vi "SFC_Get Hang Carton.vi"(8 "error in (no error)":errorcluster caption="错误输入（无错误）", 11 "Traceability 引用句柄":refnum<k24>) -> (0 "error out":errorcluster caption="错误输出", 2 ".NET:System.Data.DataSet":T1={"CaseSensitive"=FALSE, "Container"=refnum, "DataSetName"="", "DefaultViewManager"=refnum, "DesignMode"=FALSE, "EnforceConstraints"=FALSE, "ExtendedProperties"=refnum, "HasErrors"=FALSE, "IsInitialized"=FALSE, "Locale"=refnum, "Namespace"="", "Prefix"="", "Relations"=refnum, "RemotingFormat"=0, "SchemaSerializationMode"=1, "Site"=refnum, "Tables"=refnum} {"SchemaSerializationMode" items=["IncludeSchema"=1, "ExcludeSchema"=2]; "RemotingFormat" items=["Xml", "Binary"]}, 3 "Traceability 引用句柄输出":refnum<k24>)   [LabVIEW 2014, in "Traceability.lvlib"]
uses:
  D:/webservice/Traceability.dll
  Traceability.dll
  System.Data
  Traceability.lvlib
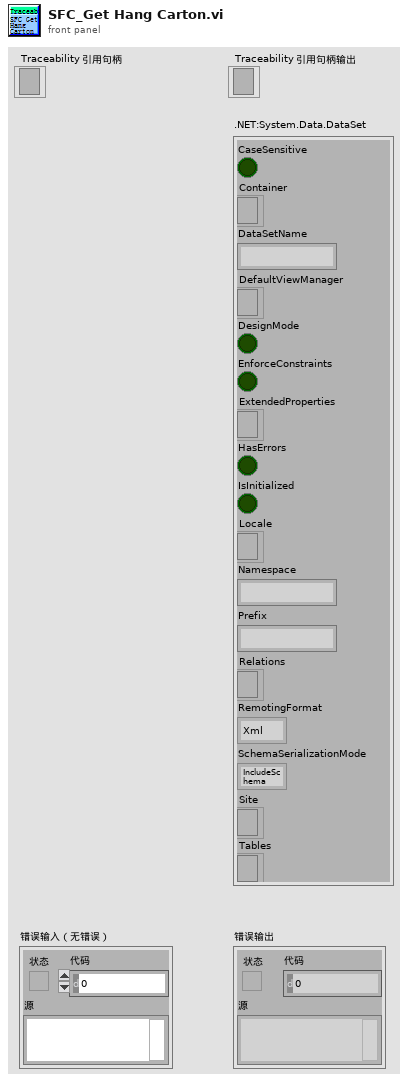
[diagram p1: front panel]
types:
  T1 = cluster{"CaseSensitive":bool, "Container":refnum<k24>, "DataSetName":string, "DefaultViewManager":refnum<k24>, "DesignMode":bool, "EnforceConstraints":bool, "ExtendedProperties":refnum<k24>, "HasErrors":bool, "IsInitialized":bool, "Locale":refnum<k24>, "Namespace":string, "Prefix":string, "Relations":refnum<k24>, "RemotingFormat":i32, "SchemaSerializationMode":i32, "Site":refnum<k24>, "Tables":refnum<k24>}
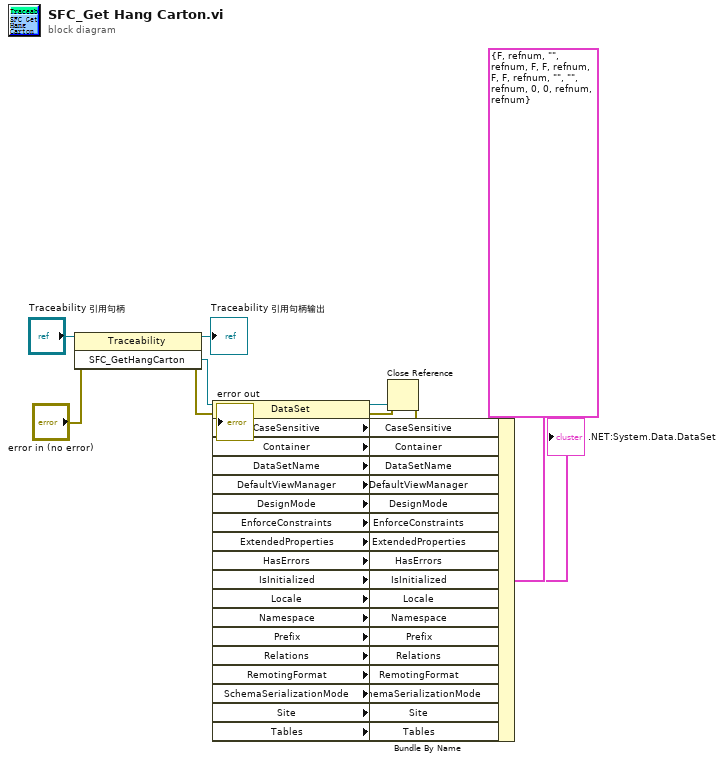
[diagram p0: block diagram]
diagram:
  n1 = invoke class="Traceability" method="SFC_GetHangCarton"(reference="Traceability 引用句柄", error in="error in (no error)") -> (reference out=→"Traceability 引用句柄输出":refnum<k24>, error out=w4:errorcluster, "SFC_GetHangCarton"=w24:refnum<k24>)  [unwired: 1 in]
  n2 = property class="DataSet"(reference=w24, error in=w4) -> (reference out=w3:refnum<k24>, error out=w2:errorcluster, "CaseSensitive"=w21:bool, "Container"=w20:refnum<k24>, "DataSetName"=w19:string, "DefaultViewManager"=w18:refnum<k24>, "DesignMode"=w17:bool, "EnforceConstraints"=w16:bool, "ExtendedProperties"=w15:refnum<k24>, "HasErrors"=w14:bool, "IsInitialized"=w13:bool, "Locale"=w12:refnum<k24>, "Namespace"=w11:string, "Prefix"=w10:string, "Relations"=w9:refnum<k24>, "RemotingFormat"=w8:i32, "SchemaSerializationMode"=w7:i32, "Site"=w6:refnum<k24>, "Tables"=w5:refnum<k24>)
  n3 = Bundle By Name(cluster=T1 {"CaseSensitive"=FALSE, "Container"=refnum, "DataSetName"="", "DefaultViewManager"=refnum, "DesignMode"=FALSE, "EnforceConstraints"=FALSE, "ExtendedProperties"=refnum, "HasErrors"=FALSE, "IsInitialized"=FALSE, "Locale"=refnum, "Namespace"="", "Prefix"="", "Relations"=refnum, "RemotingFormat"=0, "SchemaSerializationMode"=0, "Site"=refnum, "Tables"=refnum} (".NET:System.Data.DataSet"), "CaseSensitive"=w21, "Container"=w20, "DataSetName"=w19, "DefaultViewManager"=w18, "DesignMode"=w17, "EnforceConstraints"=w16, "ExtendedProperties"=w15, "HasErrors"=w14, "IsInitialized"=w13, "Locale"=w12, "Namespace"=w11, "Prefix"=w10, "Relations"=w9, "RemotingFormat"=w8, "SchemaSerializationMode"=w7, "Site"=w6, "Tables"=w5) -> (→".NET:System.Data.DataSet":T1)
  n4 = Close Reference(reference=w3, error in (no error)=w2) -> (error out=→"error out":errorcluster)
